vi "Interact with Subprocess.vi"(5 "id to check":u32, 6 "deadline":T1={"mode"=enum."Relative", "deadline (ms)"=30000}, 7 "check id":bool=TRUE, 8 "error in":errorcluster, 11 "connection in":refnum<class "Low Level Connection.lvclass">) -> (0 "error out":errorcluster, 3 "connection out":refnum<class "Low Level Connection.lvclass">)   [LabVIEW 2020, in "NI_SFTP.lvlib" / "Low Level Connection.lvclass"]
uses:
  <vilib>/net/SFTP/Low Level Connection/Low Level Connection.lvclass
  <vilib>/Utility/Deadline/Deadline.ctl
  <vilib>/Utility/Deadline/Mode.ctl
  <vilib>/net/SFTP/Low Level Connection/Low Level Connection.lvclass/Low Level Connection.ctl
  <vilib>/Array/Bytestream/Bytestream.lvclass/Bytestream.ctl
  <vilib>/Array/Bytestream/Get Logical Datum.vi
  <vilib>/Array/Bytestream/Datum Size.vi
  <vilib>/Array/Bytestream/Count Datums.vi
  <vilib>/Subprocess/Buffered Subprocess/Buffered Subprocess.lvclass
  <vilib>/Array/Bytestream/Bytestream.lvclass
  <vilib>/Utility/Deadline/NI_Deadline.lvlib
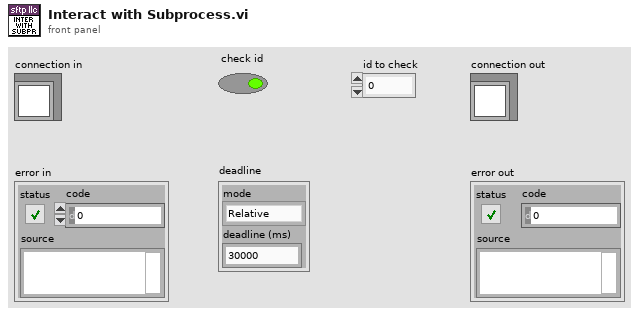
[diagram p1: front panel]
types:
  T1 = typedef "NI_Deadline.lvlib/Deadline.ctl" = cluster{"mode":T2, "deadline (ms)":u32}
  T2 = typedef "NI_Deadline.lvlib/Mode.ctl" = enum16{"Relative", "Use deadline", "Wait forever", "Nonblocking", "N/A"}
  T3 = typedef "NI_SFTP.lvlib/Low Level Connection.lvclass/Receive Map.ctl" = map{u32, T4}
  T4 = typedef "NI_SFTP.lvlib/Low Level Connection.lvclass/Packet.ctl" = cluster{"Type":T5, "payload":u8[]}
  T5 = typedef "NI_SFTP.lvlib/Low Level Connection.lvclass/Packet Type.ctl" = enum16{"SSH_FXP_TYPE_000", "SSH_FXP_INIT", "SSH_FXP_VERSION", "SSH_FXP_OPEN", "SSH_FXP_CLOSE", "SSH_FXP_READ", "SSH_FXP_WRITE", "SSH_FXP_LSTAT", "SSH_FXP_FSTAT", "SSH_FXP_SETSTAT", "SSH_FXP_FSETSTAT", "SSH_FXP_OPENDIR", "SSH_FXP_READDIR", "SSH_FXP_REMOVE", "SSH_FXP_MKDIR", "SSH_FXP_RMDIR", "SSH_FXP_REALPATH", "SSH_FXP_STAT", "SSH_FXP_RENAME", "SSH_FXP_READLINK", "SSH_FXP_SYMLINK", "SSH_FXP_LINK", "SSH_FXP_BLOCK", "SSH_FXP_UNBLOCK", "SSH_FXP_TYPE_024", "SSH_FXP_TYPE_025", "SSH_FXP_TYPE_026", "SSH_FXP_TYPE_027", "SSH_FXP_TYPE_028", "SSH_FXP_TYPE_029", "SSH_FXP_TYPE_030", "SSH_FXP_TYPE_031", "SSH_FXP_TYPE_032", "SSH_FXP_TYPE_033", "SSH_FXP_TYPE_034", "SSH_FXP_TYPE_035", "SSH_FXP_TYPE_036", "SSH_FXP_TYPE_037", "SSH_FXP_TYPE_038", "SSH_FXP_TYPE_039", "SSH_FXP_TYPE_040", "SSH_FXP_TYPE_041", "SSH_FXP_TYPE_042", "SSH_FXP_TYPE_043", "SSH_FXP_TYPE_044", "SSH_FXP_TYPE_045", "SSH_FXP_TYPE_046", "SSH_FXP_TYPE_047", "SSH_FXP_TYPE_048", "SSH_FXP_TYPE_049", "SSH_FXP_TYPE_050", "SSH_FXP_TYPE_051", "SSH_FXP_TYPE_052", "SSH_FXP_TYPE_053", "SSH_FXP_TYPE_054", "SSH_FXP_TYPE_055", "SSH_FXP_TYPE_056", "SSH_FXP_TYPE_057", "SSH_FXP_TYPE_058", "SSH_FXP_TYPE_059", "SSH_FXP_TYPE_060", "SSH_FXP_TYPE_061", "SSH_FXP_TYPE_062", "SSH_FXP_TYPE_063", "SSH_FXP_TYPE_064", "SSH_FXP_TYPE_065", "SSH_FXP_TYPE_066", "SSH_FXP_TYPE_067", "SSH_FXP_TYPE_068", "SSH_FXP_TYPE_069", "SSH_FXP_TYPE_070", "SSH_FXP_TYPE_071", "SSH_FXP_TYPE_072", "SSH_FXP_TYPE_073", "SSH_FXP_TYPE_074", "SSH_FXP_TYPE_075", "SSH_FXP_TYPE_076", "SSH_FXP_TYPE_077", "SSH_FXP_TYPE_078", "SSH_FXP_TYPE_079", "SSH_FXP_TYPE_080", "SSH_FXP_TYPE_081", "SSH_FXP_TYPE_082", "SSH_FXP_TYPE_083", "SSH_FXP_TYPE_084", "SSH_FXP_TYPE_085", "SSH_FXP_TYPE_086", "SSH_FXP_TYPE_087", "SSH_FXP_TYPE_088", "SSH_FXP_TYPE_089", "SSH_FXP_TYPE_090", "SSH_FXP_TYPE_091", "SSH_FXP_TYPE_092", "SSH_FXP_TYPE_093", "SSH_FXP_TYPE_094", "SSH_FXP_TYPE_095", "SSH_FXP_TYPE_096", "SSH_FXP_TYPE_097", "SSH_FXP_TYPE_098", "SSH_FXP_TYPE_099", "SSH_FXP_TYPE_100", "SSH_FXP_STATUS", "SSH_FXP_HANDLE", "SSH_FXP_DATA", "SSH_FXP_NAME", "SSH_FXP_ATTRS", "SSH_FXP_TYPE_106", "SSH_FXP_TYPE_107", "SSH_FXP_TYPE_108", "SSH_FXP_TYPE_109", "SSH_FXP_TYPE_110", "SSH_FXP_TYPE_111", "SSH_FXP_TYPE_112", "SSH_FXP_TYPE_113", "SSH_FXP_TYPE_114", "SSH_FXP_TYPE_115", "SSH_FXP_TYPE_116", "SSH_FXP_TYPE_117", "SSH_FXP_TYPE_118", "SSH_FXP_TYPE_119", "SSH_FXP_TYPE_120", "SSH_FXP_TYPE_121", "SSH_FXP_TYPE_122", "SSH_FXP_TYPE_123", "SSH_FXP_TYPE_124", "SSH_FXP_TYPE_125", "SSH_FXP_TYPE_126", "SSH_FXP_TYPE_127", "SSH_FXP_TYPE_128", "SSH_FXP_TYPE_129", "SSH_FXP_TYPE_130", "SSH_FXP_TYPE_131", "SSH_FXP_TYPE_132", "SSH_FXP_TYPE_133", "SSH_FXP_TYPE_134", "SSH_FXP_TYPE_135", "SSH_FXP_TYPE_136", "SSH_FXP_TYPE_137", "SSH_FXP_TYPE_138", "SSH_FXP_TYPE_139", "SSH_FXP_TYPE_140", "SSH_FXP_TYPE_141", "SSH_FXP_TYPE_142", "SSH_FXP_TYPE_143", "SSH_FXP_TYPE_144", "SSH_FXP_TYPE_145", "SSH_FXP_TYPE_146", "SSH_FXP_TYPE_147", "SSH_FXP_TYPE_148", "SSH_FXP_TYPE_149", "SSH_FXP_TYPE_150", "SSH_FXP_TYPE_151", "SSH_FXP_TYPE_152", "SSH_FXP_TYPE_153", "SSH_FXP_TYPE_154", "SSH_FXP_TYPE_155", "SSH_FXP_TYPE_156", "SSH_FXP_TYPE_157", "SSH_FXP_TYPE_158", "SSH_FXP_TYPE_159", "SSH_FXP_TYPE_160", "SSH_FXP_TYPE_161", "SSH_FXP_TYPE_162", "SSH_FXP_TYPE_163", "SSH_FXP_TYPE_164", "SSH_FXP_TYPE_165", "SSH_FXP_TYPE_166", "SSH_FXP_TYPE_167", "SSH_FXP_TYPE_168", "SSH_FXP_TYPE_169", "SSH_FXP_TYPE_170", "SSH_FXP_TYPE_171", "SSH_FXP_TYPE_172", "SSH_FXP_TYPE_173", "SSH_FXP_TYPE_174", "SSH_FXP_TYPE_175", "SSH_FXP_TYPE_176", "SSH_FXP_TYPE_177", "SSH_FXP_TYPE_178", "SSH_FXP_TYPE_179", "SSH_FXP_TYPE_180", "SSH_FXP_TYPE_181", "SSH_FXP_TYPE_182", "SSH_FXP_TYPE_183", "SSH_FXP_TYPE_184", "SSH_FXP_TYPE_185", "SSH_FXP_TYPE_186", "SSH_FXP_TYPE_187", "SSH_FXP_TYPE_188", "SSH_FXP_TYPE_189", "SSH_FXP_TYPE_190", "SSH_FXP_TYPE_191", "SSH_FXP_TYPE_192", "SSH_FXP_TYPE_193", "SSH_FXP_TYPE_194", "SSH_FXP_TYPE_195", "SSH_FXP_TYPE_196", "SSH_FXP_TYPE_197", "SSH_FXP_TYPE_198", "SSH_FXP_TYPE_199", "SSH_FXP_EXTENDED", "SSH_FXP_EXTENDED_REPLY"}
  T6 = cluster{"subprocess":refnum<class "Buffered Subprocess.lvclass">, "read stdout":refnum<class "Bytestream.lvclass">}
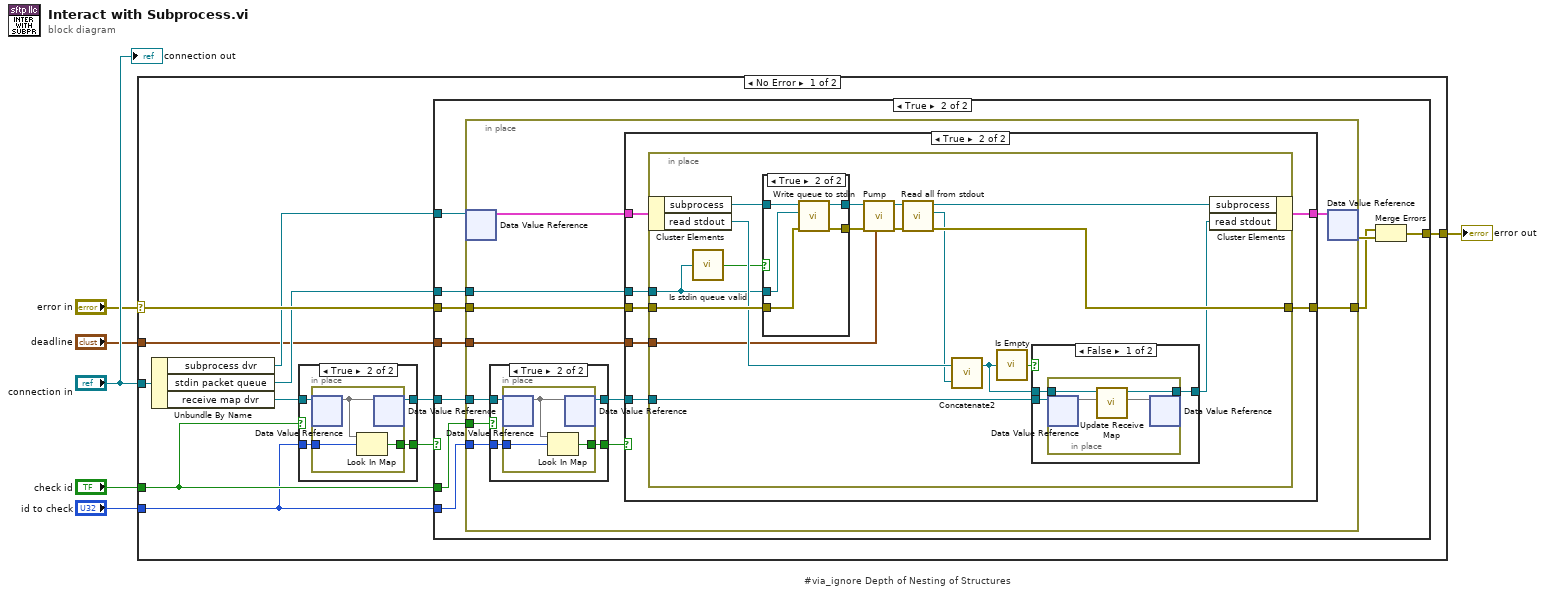
[diagram p0: block diagram]
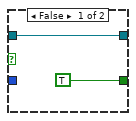
[diagram p6: hidden frame]
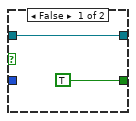
[diagram p7: hidden frame]
diagram:
  # "#via_ignore Depth of Nesting of Structures"
  n1 = case shown="No Error" "error in" {
    selector: "error in" -> [w13 w98]
    tunnel: [w17 w98] -> w6
    tunnel: "check id" -> [w16 _]
    tunnel: "id to check" -> [w15 _]
    tunnel: "connection in" -> [w14 _]
    tunnel: "deadline" -> [w7 _]
    frame No Error {
      n2 = Unbundle By Name(w14) -> ("subprocess dvr"=w10:refnum<data-value>, "stdin packet queue"=w9:refnum<queue>, "receive map dvr"=w11:refnum<data-value>)
      n3 = case shown="True" w16 {
        tunnel: w15 -> [_ w94]
        tunnel: w11 -> [w89 w93]
        tunnel: [TRUE ("key not found?") w92] -> w12
        tunnel: [w89 w91] -> w8
        frame False {
        }
        frame True {
          n4 = in-place {
            in-place-border: w94 -> [w97]
            in-place-border: [w96] -> w92
            n5 = in-place-dvr #1(w93) -> (w95:T3)  [unwired: 1 out]
            n6 = Look In Map(map=w95, key=w97) -> (key not found?=w96:bool)  [unwired: 1 in, 1 out]
            n7 = in-place-dvr #1(w95) -> (w91:refnum<data-value>)  [unwired: 1 out]
          }
        }
      }
      n8 = case shown="True" w12 {
        tunnel: w13 -> [w18 w26]
        tunnel: [w18 w20] -> w17
        tunnel: w16 -> [_ w23]
        tunnel: w15 -> [_ w24]
        tunnel: w10 -> [_ w28]
        tunnel: w9 -> [_ w27]
        tunnel: w8 -> [_ w25]
        tunnel: w7 -> [_ w19]
        frame False {
        }
        frame True {
          n9 = in-place {
            in-place-border: w26 -> [w37]
            in-place-border: [w39] -> w21
            in-place-border: w27 -> [w38]
            in-place-border: w23 -> [w34]
            in-place-border: w24 -> [w33]
            in-place-border: w25 -> [w32]
            in-place-border: w19 -> [w29]
            n10 = in-place-dvr #2(w28) -> (w36:T6)  [unwired: 1 out]
            n11 = case shown="True" w34 {
              tunnel: w33 -> [_ w85]
              tunnel: w32 -> [w81 w84]
              tunnel: [w81 w83] -> w31
              tunnel: [TRUE ("key not found?") w82] -> w30
              frame False {
              }
              frame True {
                n12 = in-place {
                  in-place-border: w85 -> [w88]
                  in-place-border: [w87] -> w82
                  n13 = in-place-dvr #3(w84) -> (w86:T3)  [unwired: 1 out]
                  n14 = Look In Map(map=w86, key=w88) -> (key not found?=w87:bool)  [unwired: 1 in, 1 out]
                  n15 = in-place-dvr #3(w86) -> (w83:refnum<data-value>)  [unwired: 1 out]
                }
              }
            }
            n16 = case shown="True" w30 {
              tunnel: [w41 w48] -> w39
              tunnel: w38 -> [_ w47]
              tunnel: w37 -> [w41 w46]
              tunnel: w36 -> [w40 w45]
              tunnel: [w40 w44] -> w35
              tunnel: w31 -> [_ w43]
              tunnel: w29 -> [_ w42]
              frame False {
              }
              frame True {
                n17 = in-place {
                  in-place-border: [w64] -> w48
                  in-place-border: w47 -> [w50]
                  in-place-border: w46 -> [w63]
                  in-place-border: w43 -> [w62]
                  in-place-border: w42 -> [w51]
                  n18 = in-place-cluster #4(w45) -> ("subprocess"=w61:refnum<class "Buffered Subprocess.lvclass">, "read stdout"=w60:refnum<class "Bytestream.lvclass">)
                  n19 = call <vilib>:"Is stdin queue valid.vi"("stdin packet queue"=w50) -> ("valid?"=w49:bool)
                  n20 = case shown="True" w49 {
                    tunnel: w50 -> [_ w69]
                    tunnel: w63 -> [w65 w71]
                    tunnel: w61 -> [w66 w70]
                    tunnel: [w66 w68] -> w57
                    tunnel: [w65 w67] -> w56
                    frame False {
                    }
                    frame True {
                      n21 = call <vilib>:"Write queue to stdin.vi"("error in (no error)"=w71, "queue in"=w69, "subprocess in"=w70) -> ("error out"=w67:errorcluster, "subprocess out"=w68:refnum<class "Buffered Subprocess.lvclass">)  [unwired: 6 in, 1 out]
                    }
                  }
                  n22 = call <vilib>:"Pump.vi"("deadline"=w51, "error in (no error)"=w56, "subprocess in"=w57) -> ("error out"=w64:errorcluster, "subprocess out"=w55:refnum<class "Buffered Subprocess.lvclass">)  [unwired: 7 in]
                  n23 = call <vilib>:"Read all from stdout.vi"("subprocess in"=w55) -> ("data"=w52:refnum<class "Bytestream.lvclass">, "subprocess out"=w59:refnum<class "Buffered Subprocess.lvclass">)  [unwired: 9 in]
                  n24 = call <vilib>:"Concatenate2.vi"("b"=w52, "a"=w60) -> ("c"=w53:refnum<class "Bytestream.lvclass">)  [unwired: 1 out]
                  n25 = call <vilib>:"Is Empty.vi"("a"=w53) -> ("empty?"=w54:bool)
                  n26 = case shown="False" w54 {
                    tunnel: w62 -> [w74 _]
                    tunnel: w53 -> [w73 w79]
                    tunnel: [w72 w79] -> w58
                    frame False {
                      n27 = in-place {
                        in-place-border: w73 -> [w78]
                        in-place-border: [w75] -> w72
                        n28 = in-place-dvr #5(w74) -> (w77:T3)  [unwired: 1 out]
                        n29 = call <vilib>:"Update Receive Map.vi"("receive map"=w77, "bytestream"=w78) -> ("receive map out"=w76:map{u32, T4}, "bytestream out"=w75:refnum<class "Bytestream.lvclass">)  [unwired: 7 in, 1 out]
                        n30 = in-place-dvr #5(w76) -> ()  [unwired: 2 out]
                      }
                    }
                    frame True {
                    }
                  }
                  n31 = in-place-cluster #4("subprocess"=w59, "read stdout"=w58) -> (w44:T6)
                }
              }
            }
            n32 = in-place-dvr #2(w35) -> (w22:errorcluster)  [unwired: 1 out]
          }
          n33 = Merge Errors(w21, w22) -> (w20:errorcluster)
        }
      }
    }
    frame Error {
    }
  }
  "error out" <- w6
  "connection out" <- "connection in"
